vi "8 - CSV Ingest.vi"() -> ()   [LabVIEW 2020]
uses:
  client/client.lvlib
panel:
  out "channel list":string[](array[string])
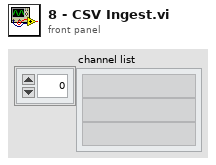
[diagram p1: front panel]
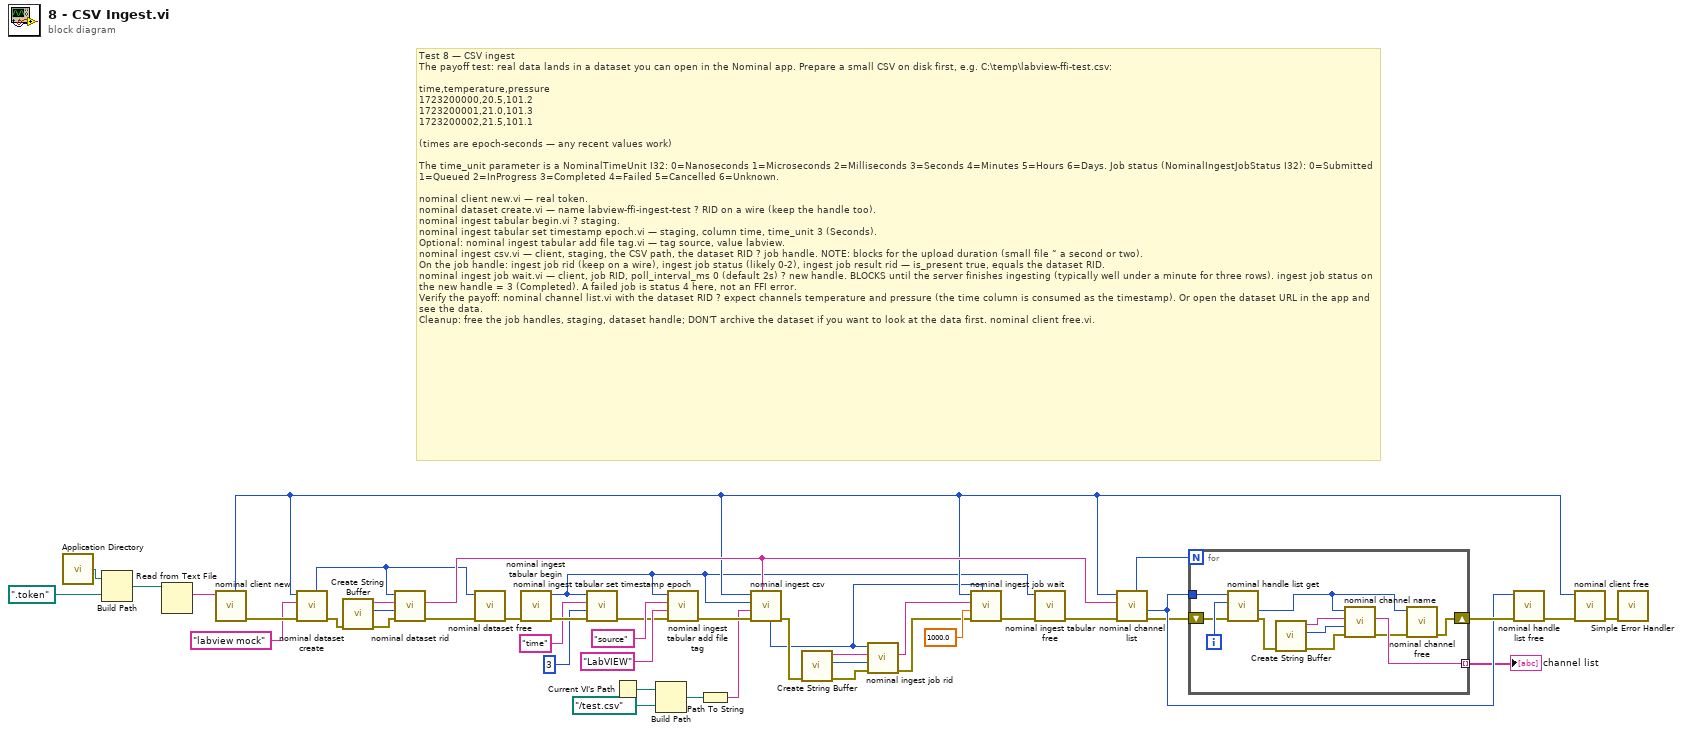
[diagram p0: block diagram]
diagram:
  # "Test 8 — CSV ingest\nThe payoff test: real data lands in a dataset you can open in the Nominal app. Prepare a small CSV on disk first, e.g. C:\\temp\\labview-ffi-test.csv:\n\ntime,temperature,pressure\n1723200000,20.5,101.2\n1723200001,21.0,101.3\n1723200002,21.5,101.1\n\n(times are epoch-seconds — any recent values work)\n\nThe time_unit parameter is a NominalTimeUnit I32: 0=Nanoseconds 1=Microseconds 2=Milliseconds 3=Seconds 4=Minutes 5=Hours 6=Days. Job status (NominalIngestJobStatus I32): 0=Submitted 1=Queued 2=InProgress 3=Completed 4=Failed 5=Cancelled 6=Unknown.\n\nnominal client new.vi — real token.\nnominal dataset create.vi — name labview-ffi-ingest-test ? RID on a wire (keep the handle too).\nnominal ingest tabular begin.vi ? staging.\nnominal ingest tabular set timestamp epoch.vi — staging, column time, time_unit 3 (Seconds).\nOptional: nominal ingest tabular add file tag.vi — tag source, value labview.\nnominal ingest csv.vi — client, staging, the CSV path, the dataset RID ? job handle. NOTE: blocks for the upload duration (small file ˜ a second or two).\nOn the job handle: ingest job rid (keep on a wire), ingest job status (likely 0-2), ingest job result rid — is_present true, equals the dataset RID.\nnominal ingest job wait.vi — client, job RID, poll_interval_ms 0 (default 2s) ? new handle. BLOCKS until the server finishes ingesting (typically well under a minute for three rows). ingest job status on the new handle = 3 (Completed). A failed job is status 4 here, not an FFI error.\nVerify the payoff: nominal channel list.vi with the dataset RID ? expect channels temperature and pressure (the time column is consumed as the timestamp). Or open the dataset URL in the app and see the data.\nCleanup: free the job handles, staging, dataset handle; DON'T archive the dataset if you want to look at the data first. nominal client free.vi."
  n1 = call <vilib>:"Application Directory.vi"() -> ("Application Directory"=w43:path)
  n2 = Build Path(base path=w43, name or relative path=path ".token") -> (appended path=w41:path)
  n3 = Read from Text File(file (use dialog)=w41) -> (text=w40:string)  [unwired: 3 in, 3 out]
  n4 = call "nominal client new.vi"("token"=w40) -> ("error out"=w39:errorcluster, "out_client out"=w18:i32)  [unwired: 8 in, 1 out]
  n5 = call "nominal dataset create.vi"("error in (no error)"=w39, "name"="labview mock", "client"=w18) -> ("error out"=w32:errorcluster, "out_dataset out"=w12:i32)  [unwired: 6 in, 1 out]
  n6 = call "Create String Buffer.vi"("error in"=w32) -> ("error out"=w33:errorcluster, "dub Buffer Size"=w34:i32, "String Buffer"=w35:string)  [unwired: 8 in]
  n7 = call "nominal dataset rid.vi"("error in (no error)"=w33, "cap"=w34, "buf"=w35, "dataset"=w12) -> ("error out"=w11:errorcluster, "buf out"=w19:string)  [unwired: 4 in, 2 out]
  n8 = call "nominal dataset free.vi"("error in (no error)"=w11, "dataset"=w12) -> ("error out"=w10:errorcluster)  [unwired: 8 in, 1 out]
  n9 = call "nominal ingest tabular begin.vi"("error in (no error)"=w10) -> ("error out"=w31:errorcluster, "out_staging out"=w13:i32)  [unwired: 8 in, 1 out]
  n10 = call "nominal ingest tabular set timestamp epoch.vi"("error in (no error)"=w31, "time_unit"=3, "column"="time", "staging"=w13) -> ("error out"=w26:errorcluster)  [unwired: 6 in, 1 out]
  n11 = Current VI's Path() -> (path=w24:path)
  n12 = Build Path(base path=w24, name or relative path=path "../test.csv") -> (appended path=w22:path)
  n13 = call "nominal ingest tabular add file tag.vi"("error in (no error)"=w26, "value"="LabVIEW" ("tag"), "tag"="source", "staging"=w13) -> ("error out"=w25:errorcluster)  [unwired: 6 in, 1 out]
  n14 = Path To String(path=w22) -> (string=w21:string)
  n15 = call "nominal ingest csv.vi"("dataset_rid"=w19, "error in (no error)"=w25, "file_path"=w21, "staging"=w13, "client"=w18) -> ("error out"=w7:errorcluster, "out_job out"=w2:i32)  [unwired: 4 in, 1 out]
  n16 = call "Create String Buffer.vi"("error in"=w7) -> ("error out"=w8:errorcluster, "dub Buffer Size"=w3:i32, "String Buffer"=w9:string)  [unwired: 8 in]
  n17 = call "nominal ingest job rid.vi"("error in (no error)"=w8, "cap"=w3, "buf"=w9, "job"=w2) -> ("error out"=w5:errorcluster, "buf out"=w6:string)  [unwired: 4 in, 2 out]
  n18 = call "nominal ingest job wait.vi"("out_job"=w2, "error in (no error)"=w5, "poll_interval_ms"=1000.0, "rid"=w6, "client"=w18) -> ("error out"=w4:errorcluster)  [unwired: 4 in, 2 out]
  n19 = call "nominal ingest tabular free.vi"("error in (no error)"=w4, "staging"=w13) -> ("error out"=w1:errorcluster)  [unwired: 8 in, 1 out]
  n20 = call "nominal channel list.vi"("error in (no error)"=w1, "data_source_rid"=w19, "client"=w18) -> ("error out"=w15:errorcluster, "out_list out"=w16:i32, "out_count out"=w17:u32)  [unwired: 5 in, 1 out]
  n21 = for {
    N: w17 -> [_]
    tunnel: w16 -> [w55]
    shift-right: [w46] -> w37
    shift-left: w15 -> [w53]
    tunnel: [w48] -> w14 mode=indexing
    i -> [w54]
    n22 = call "nominal handle list get.vi"("error in (no error)"=w53, "index"=w54, "list"=w55) -> ("error out"=w52:errorcluster, "out_handle out"=w45:i32)  [unwired: 6 in, 1 out]
    n23 = call "Create String Buffer.vi"("error in"=w52) -> ("error out"=w51:errorcluster, "dub Buffer Size"=w50:i32, "String Buffer"=w49:string)  [unwired: 8 in]
    n24 = call "nominal channel name.vi"("error in (no error)"=w51, "cap"=w50, "buf"=w49, "channel"=w45) -> ("error out"=w47:errorcluster, "buf out"=w48:string)  [unwired: 4 in, 2 out]
    n25 = call "nominal channel free.vi"("error in (no error)"=w47, "channel"=w45) -> ("error out"=w46:errorcluster)  [unwired: 8 in, 1 out]
  }
  "channel list" <- w14
  n26 = call "nominal handle list free.vi"("error in (no error)"=w37, "list"=w16) -> ("error out"=w36:errorcluster)  [unwired: 8 in, 1 out]
  n27 = call "nominal client free.vi"("error in (no error)"=w36, "client"=w18) -> ("error out"=w44:errorcluster)  [unwired: 8 in, 1 out]
  n28 = call <vilib>:"Simple Error Handler.vi"("error in (no error)"=w44) -> ()  [unwired: 4 in, 5 out]
